vi "Load calibration profile data file.vi"(8 "error in (no error)":errorcluster, 11 "Path":path) -> (0 "error out":errorcluster, 2 "Column Headers":string[][](array[string]), 3 "Data":string[][](array[string]), 5 "File Name":string)   [LabVIEW 2020]
panel:
  out "Array":string[][](array[string])
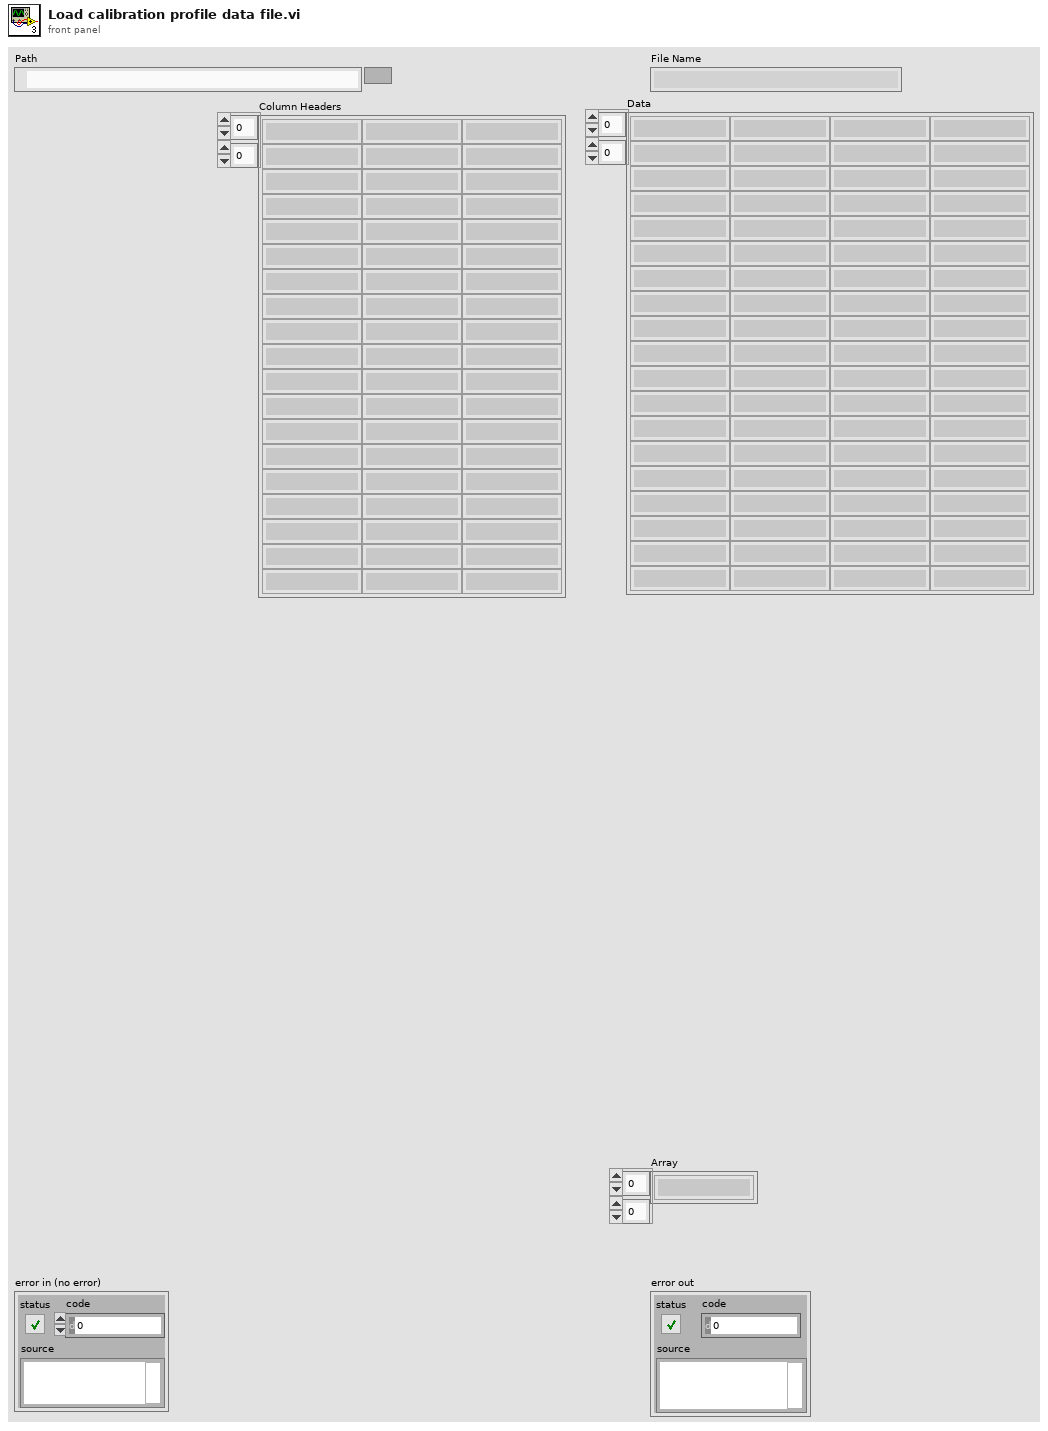
[diagram p1: front panel]
types:
  T1 = enum16{"open", "replace", "create", "open or create", "replace or create", "replace or create with confirmation"}
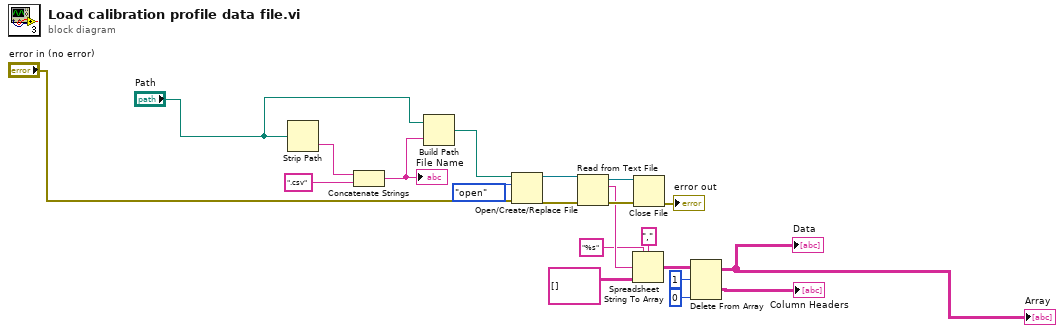
[diagram p0: block diagram]
diagram:
  n1 = Strip Path(path="Path") -> (name=w1:string)  [unwired: 1 out]
  n2 = Concatenate Strings(w1, ".csv" ("string")) -> (w15:string)
  "File Name" <- w15
  n3 = Build Path(base path="Path", name or relative path=w15) -> (appended path=w4:path)
  n4 = Open/Create/Replace File(file path (use dialog)=w4, error in="error in (no error)", operation (0:open)=T1."open") -> (refnum out=w7:refnum<file>, error out=w6:errorcluster)  [unwired: 3 in, 1 out]
  n5 = Read from Text File(file (use dialog)=w7, error in=w6) -> (refnum out=w13:refnum<file>, text=w11:string, error out=w12:errorcluster)  [unwired: 2 in, 1 out]
  n6 = Spreadsheet String To Array(delimiter (Tab)=",", format string="%s", spreadsheet string=w11, array type (2D Dbl)=string[][] []) -> (array=w16:string[][])
  n7 = Close File(refnum=w13, error in=w12) -> (error out=→"error out":errorcluster)  [unwired: 1 out]
  n8 = Delete From Array(array=w16, length=1, index (row)=0) -> (deleted portion=→"Column Headers":string[][], array with subset deleted=→"Data" →"Array":string[][])  [unwired: 1 in]
